vi "data to datatable.vi"(9 "dis config Array":T1(array[cluster]), 11 "CalData":T2(array[cluster])) -> (3 "datatable":string[][](array[string]))   [LabVIEW 2011]
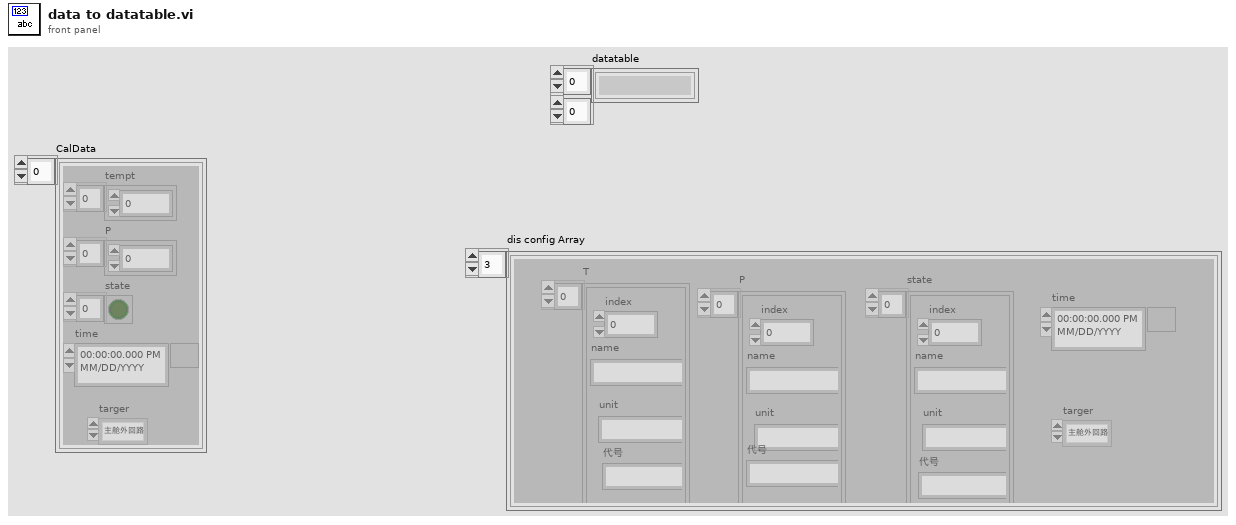
[diagram p1: front panel]
types:
  T1 = cluster{"T":cluster{"index":dbl, "name":string, "unit":string, "代号":string}[], "P":cluster{"index":dbl, "name":string, "unit":string, "代号":string}[], "state":cluster{"index":dbl, "name":string, "unit":string, "代号":string}[], "time":timestamp, "targer":enum16{"主舱外回路", "主舱内回路", "实验舱外回路", "实验舱内回路"}}[]
  T2 = cluster{"tempt":dbl[], "P":dbl[], "state":bool[], "time":timestamp, "targer":enum16{"主舱外回路", "主舱内回路", "实验舱外回路", "实验舱内回路"}}[]
  T3 = cluster{"tempt":dbl[], "P":dbl[], "state":bool[], "time":timestamp, "targer":enum16{"主舱外回路", "主舱内回路", "实验舱外回路", "实验舱内回路"}}
  T4 = cluster{"index":dbl, "name":string, "unit":string, "代号":string}[]
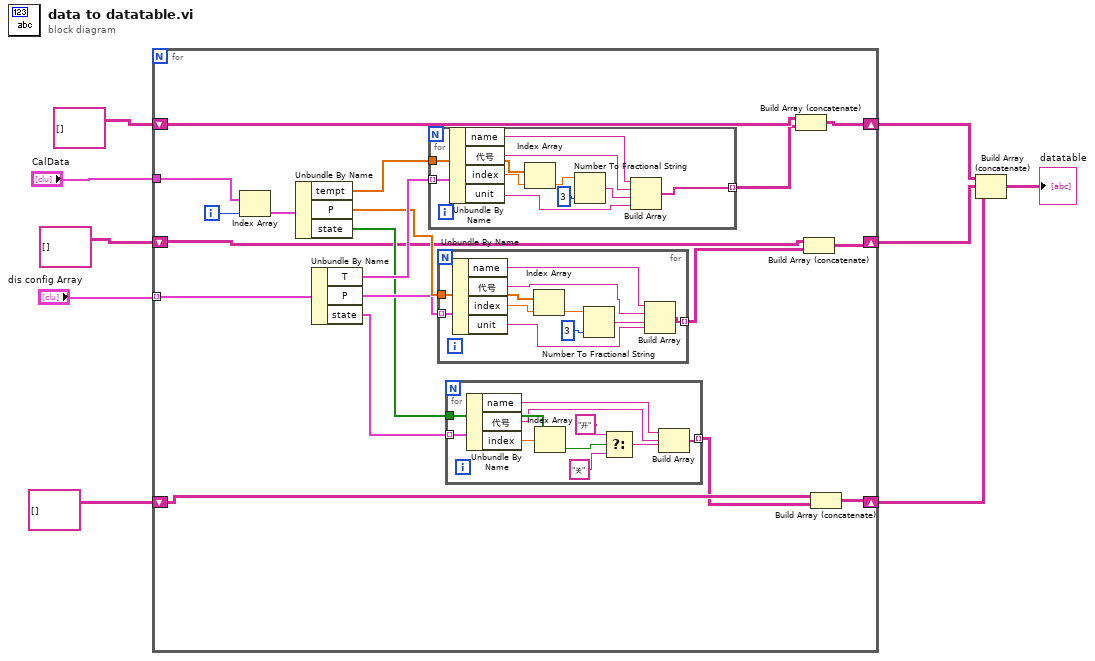
[diagram p0: block diagram]
diagram:
  n1 = for {
    tunnel: "CalData" -> [w28]
    tunnel: "dis config Array" -> [w25] mode=indexing
    shift-right: [w18] -> w4
    shift-left: string[][] [] -> [w11]
    shift-right: [w12] -> w3
    shift-left: string[][] [] -> [w13]
    shift-right: [w15] -> w2
    shift-left: string[][] [] -> [w17]
    i -> [w27]
    n2 = Index Array(array=w28, index=w27) -> (element=w26:T3)
    n3 = Unbundle By Name(w26) -> ("tempt"=w23:dbl[], "P"=w22:dbl[], "state"=w19:bool[])
    n4 = Unbundle By Name(w25) -> ("T"=w24:T4, "P"=w21:T4, "state"=w20:T4)
    n5 = for {
      tunnel: w24 -> [w58] mode=indexing
      tunnel: w23 -> [w57]
      tunnel: [w53] -> w10 mode=indexing
      n6 = Unbundle By Name(w58) -> ("name"=w50:string, "代号"=w49:string, "index"=w56:dbl, "unit"=w54:string)
      n7 = Index Array(array=w57, index=w56) -> (element=w55:dbl)
      n8 = Number To Fractional String(number=w55, precision (6)=i16 3 ("width (-)")) -> (F-format string=w51:string)  [unwired: 2 in]
      n9 = Build Array "Build Array"(w50, w49, w51, w54) -> (w53:string[])
    }
    n10 = for {
      tunnel: w21 -> [w48] mode=indexing
      tunnel: w22 -> [w47]
      tunnel: [w42] -> w14 mode=indexing
      n11 = Unbundle By Name(w48) -> ("name"=w40:string, "代号"=w39:string, "index"=w46:dbl, "unit"=w43:string)
      n12 = Index Array(array=w47, index=w46) -> (element=w45:dbl)
      n13 = Number To Fractional String(number=w45, precision (6)=i16 3 ("width (-)")) -> (F-format string=w44:string)  [unwired: 2 in]
      n14 = Build Array(w40, w39, w44, w43) -> (w42:string[])
    }
    n15 = for {
      tunnel: w20 -> [w38] mode=indexing
      tunnel: w19 -> [w37]
      tunnel: [w34] -> w16 mode=indexing
      n16 = Unbundle By Name(w38) -> ("name"=w29:string, "代号"=w35:string, "index"=w36:dbl)
      n17 = Index Array(array=w37, index=w36) -> (element=w33:bool)
      n18 = Select(t="开", s=w33, f="关") -> (s? t:f=w30:string)
      n19 = Build Array(w29, w35, w30) -> (w34:string[])
    }
    n20 = Build Array (concatenate)(w11, w10) -> (w18:string[][])
    n21 = Build Array (concatenate)(w13, w14) -> (w12:string[][])
    n22 = Build Array (concatenate)(w17, w16) -> (w15:string[][])
  }
  n23 = Build Array (concatenate)(w4, w3, w2) -> (→"datatable":string[][])
